vi "DriveExecute.vi"(8 "error in (no error)":errorcluster) -> (0 "error out":errorcluster)   [LabVIEW 2023]
doc: "Execute for Drie\n\nClosed control loop for drive\n\ninput: \n error in (cluster)\n\noutput:\n error out (cluster)"
uses:
  DriveGlobal.vi
  <vilib>/Rock Robotics/WPI/ThirdParty/JAS_Junk/TrajLib/Trajectory_Library.lvlib
  <vilib>/Rock Robotics/WPI/ThirdParty/JAS_Junk/TrajLib/LinearFilter_LP_BW1_Execute.vi
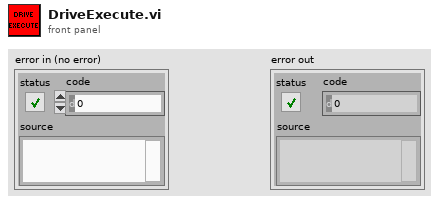
[diagram p1: front panel]
types:
  T1 = typedef "Trajectory_Library.lvlib/CHASSIS_SPEEDS.ctl" = cluster{"vX":dbl, "vY":dbl, "vOmega":dbl}
  T2 = typedef "ADIS16470 Device Reference.ctl" = cluster{"DevStatus":errorcluster, "Hardware Config":T3, "Calibration Complete":refnum<notifier>, "Status Reference":refnum<data-value>, "Data Reference":refnum<data-value>, "Sychronous Process VI":T7, "Cmd FIFO":refnum<k33>, "Source":T8, "Data FIFO":refnum<k33>, "Calibration Time (ms)":u32, "Data Reference":refnum<data-value>}
  T3 = typedef "ADIS16470 Hardware Configuration.ctl" = cluster{"SPI Clock Rate (Hz)":dbl, "IMU SPI Mode (3)":T4, "IMU Reset Pin":T5, "IMU SPI Bus":T6, "IMU Data Ready Pin":T5, "Stall Config":cluster{"Pow2BytesPerRead":u8, "StallTicks":u16, "CsToSclkTicks":u8}}
  T4 = typedef "WPI_SPIMode.ctl" = enum16{"Mode 0 (Clk Idle Low,Sample on Leading)", "Mode 1 (Clk Idle Low,Sample on Trailing)", "Mode 2 (Clk Idle High,Sample on Leading)", "Mode 3 (Clk Idle High,Sample on Trailing)"}
  T5 = typedef "FPGA_DIOChannel.ctl" = enum8{"DIO 0", "DIO 1", "DIO 2", "DIO 3", "DIO 4", "DIO 5", "DIO 6", "DIO 7", "DIO 8", "DIO 9", "DIO MXP 0", "DIO MXP 1", "DIO MXP 2", "DIO MXP 3", "DIO MXP 4", "DIO MXP 5", "DIO MXP 6", "DIO MXP 7", "DIO MXP 8", "DIO MXP 9", "DIO MXP 10", "DIO MXP 11", "DIO MXP 12", "DIO MXP 13", "DIO MXP 14", "DIO MXP 15", "SPI Port CS1", "SPI Port CS2", "SPI Port CS3", "SPI Port MISO", "SPI Port MOSI", "Invalid"}
  T6 = typedef "spi_bus.ctl" = enum16{"SPI On-Board, CS0", "SPI On-Board, CS1", "SPI On-Board, CS2", "SPI On-Board, CS3", "SPI MXP", "Invalid"}
  T7 = typedef "ADIS16470 Process.ctl" = refnum<vi>
  T8 = typedef "FPGA_CounterEncoderSourceConvertionLVSourceType.ctl" = cluster{"DevStatus":errorcluster, "AnalogTriggerMode?":bool, "DigitalMode":cluster{"DIO Channel":T9}, "AnalogTriggerMode":cluster{"AnalogTriggerIndex":T10, "OutputType":T11}}
  T9 = typedef "FPGA_DIODigitalSourceChannel.ctl" = enum8{"DIO 0", "DIO 1", "DIO 2", "DIO 3", "DIO 4", "DIO 5", "DIO 6", "DIO 7", "DIO 8", "DIO 9", "DIO MXP 0", "DIO MXP 1", "DIO MXP 2", "DIO MXP 3", "DIO MXP 4", "DIO MXP 5", "DIO MXP 6", "DIO MXP 7", "DIO MXP 8", "DIO MXP 9", "DIO MXP 10", "DIO MXP 11", "DIO MXP 12", "DIO MXP 13", "DIO MXP 14", "DIO MXP 15", "SPI Port CS1", "SPI Port CS2", "SPI Port CS3", "SPI Port MISO", "SPI Port MOSI", "Disabled"}
  T10 = typedef "FPGA_AnalogTriggerIndex.ctl" = enum8{"Trig 0", "Trig 1", "Trig 2", "Trig 3", "Trig 4", "Trig 5", "Trig 6", "Trig 7", "Invalid"}
  T11 = typedef "FPGA_AnalogTriggerOutType.ctl" = enum16{"InWindow", "TriggerState", "Rising", "Falling"}
  T12 = typedef "Trajectory_Library.lvlib/SWERVE_DRIVE_KINEMATICS.ctl" = cluster{"NumModules":i32, "InverseKinematics":T13, "ForwardKinematics":T13, "Modules":T14[], "PrevCoR":T14, "SavedModuleStates":T15[]}
  T13 = typedef "NI_Matrix.lvlib/RealMatrix.ctl" = dbl[][]
  T14 = typedef "Trajectory_Library.lvlib/TRANSLATION2D.ctl" = cluster{"X":dbl, "Y":dbl}
  T15 = typedef "Trajectory_Library.lvlib/SWERVE_DRIVE_MODULE_STATE.ctl" = cluster{"Speed":dbl, "Angle":T16}
  T16 = typedef "Trajectory_Library.lvlib/ROTATION2D.ctl" = cluster{"VALUE":dbl, "COS":dbl, "SIN":dbl}
  T17 = typedef "Trajectory_Library.lvlib/SWERVE_DRIVE_MODULE_POSITION.ctl" = cluster{"Distance":dbl, "Angle":T16, "P":bool}
  T18 = typedef "ADIS16470 Data.ctl" = cluster{"XAngle":dbl, "YAngle":dbl, "ZAngle":dbl}
  T19 = typedef "ADIS16470 Status.ctl" = cluster{"Calibrated?":bool, "IMU Detected?":bool}
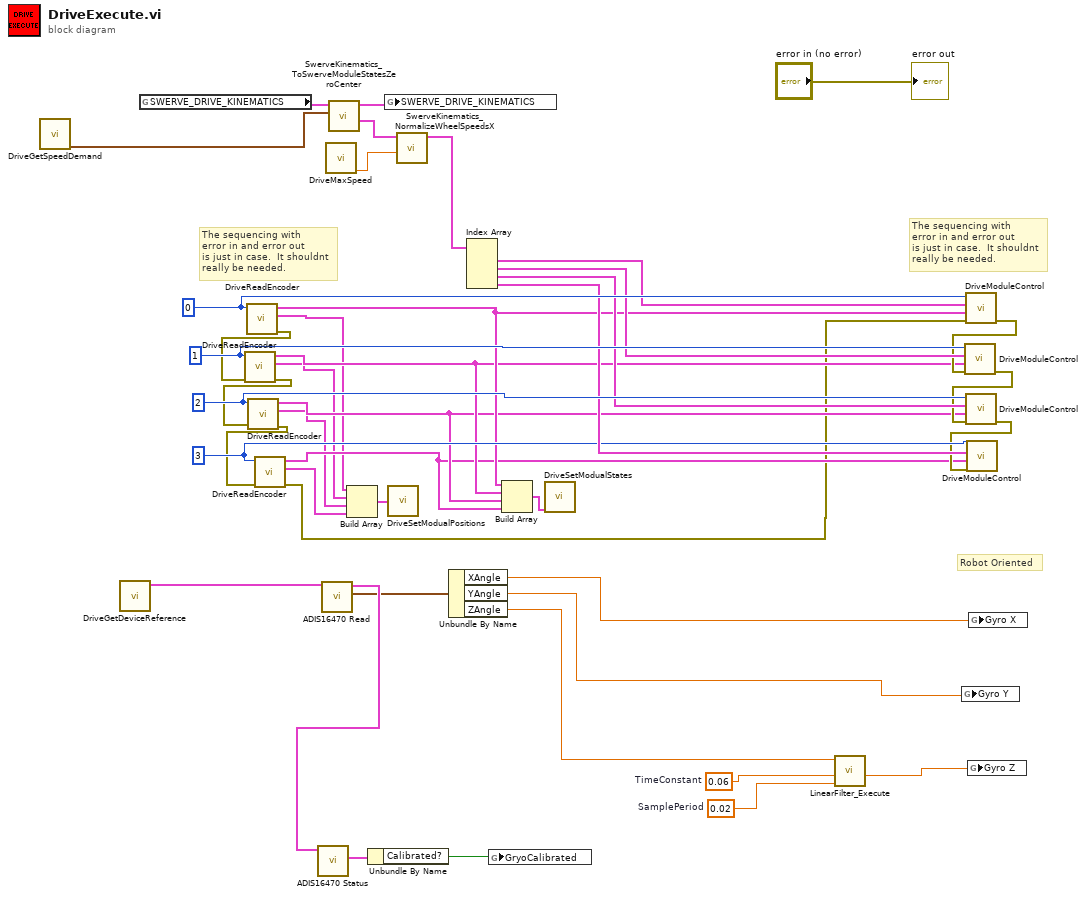
[diagram p0: block diagram]
diagram:
  w15 = 0.02  # SamplePeriod
  w1 = 0.06  # TimeConstant
  w39 = 0 ("ModualNamePrefix")
  w38 = 1 ("ModualNamePrefix")
  w37 = 2 ("ModualNamePrefix")
  w32 = 3 ("ModualNamePrefix")
  # "Robot Oriented"
  # "The sequencing with\nerror in and error out\nis just in case.  It shouldnt\nreally be needed."
  # "The sequencing with\nerror in and error out\nis just in case.  It shouldnt\nreally be needed."
  n1 = call "DriveGetSpeedDemand.vi"() -> ("ChassisSpeedDemand"=w41:T1)  [unwired: 8 in, 3 out]
  n2 = call "DriveGetDeviceReference.vi"() -> ("ADIS16470DevRef out"=w14:T2)  [unwired: 11 in]
  n3 = global read "DriveGlobal.vi" "SWERVE_DRIVE_KINEMATICS"() -> (w42:T12)
  n4 = call "DriveReadEncoder.vi"("ModualNamePrefix"=w39) -> ("error out"=w18:errorcluster, "SWERVE_DRIVE_MODULE_POSITION"=w24:T17, "SWERVE_DRIVE_MODULE_STATE"=w28:T15)  [unwired: 8 in]
  n5 = call "DriveReadEncoder.vi"("error in"=w18, "ModualNamePrefix"=w38) -> ("error out"=w17:errorcluster, "SWERVE_DRIVE_MODULE_POSITION"=w23:T17, "SWERVE_DRIVE_MODULE_STATE"=w27:T15)  [unwired: 7 in]
  n6 = call "DriveReadEncoder.vi"("error in"=w17, "ModualNamePrefix"=w37) -> ("error out"=w16:errorcluster, "SWERVE_DRIVE_MODULE_POSITION"=w22:T17, "SWERVE_DRIVE_MODULE_STATE"=w26:T15)  [unwired: 7 in]
  n7 = call "DriveReadEncoder.vi"("error in"=w16, "ModualNamePrefix"=w32) -> ("error out"=w5:errorcluster, "SWERVE_DRIVE_MODULE_POSITION"=w21:T17, "SWERVE_DRIVE_MODULE_STATE"=w25:T15)  [unwired: 7 in]
  n8 = call <vilib>:"ADIS16470 Read.vi"("ADIS16470DevRef"=w14) -> ("ADIS16470 Value"=w10:T18, "ADIS16470DevRef"=w11:T2)  [unwired: 7 in, 2 out]
  n9 = call <vilib>:"ADIS16470 Status.vi"("ADIS16470DevRef"=w11) -> ("ADIS16470 Status"=w13:T19)  [unwired: 8 in, 2 out]
  n10 = call "DriveMaxSpeed.vi"() -> ("Max Speed (m/sec)"=w3:dbl)  [unwired: 10 in, 1 out]
  n11 = call <vilib>:"SwerveKinematics_ToSwerveModuleStatesZeroCenter.vi"("ChassisSpeeds"=w41, "in SWERVE_DRIVE_KINEMATICS"=w42) -> ("ModuleStates"=w4:T15[], "out SWERVE_DRIVE_KINEMATICS"=w40:T12)  [unwired: 8 in]
  n12 = Build Array(w24, w23, w22, w21) -> (w19:T17[])
  n13 = Unbundle By Name(w13) -> ("Calibrated?"=w12:bool)
  n14 = global write "DriveGlobal.vi" "SWERVE_DRIVE_KINEMATICS"(w40) -> ()
  n15 = call "DriveSetModualPositions.vi"("Swerve_Drive_Modual_Position"=w19) -> ()  [unwired: 11 in]
  n16 = call <vilib>:"SwerveKinematics_NormalizeWheelSpeedsX.vi"("AttainableMaxSpeed"=w3, "in WheelStates"=w4) -> ("out WheelStates"=w2:T15[])  [unwired: 9 in]
  n17 = Unbundle By Name(w10) -> ("XAngle"=w8:dbl, "YAngle"=w7:dbl, "ZAngle"=w9:dbl)
  n18 = Index Array(array=w2) -> (element #1=w33:T15, element #2=w36:T15, element #3=w35:T15, element #4=w34:T15)  [unwired: 4 in]
  n19 = global write "DriveGlobal.vi" "GryoCalibrated"(w12) -> ()
  n20 = Build Array(w28, w27, w26, w25) -> (w20:T15[])
  n21 = call "DriveSetModualStates.vi"("Swerve__Drive_Modual_States"=w20) -> ()  [unwired: 11 in]
  n22 = call-poly <vilib>:"LinearFilter_Execute.vi"("SamplePeriod"=w15, "TimeConstant"=w1, "Input"=w9) -> ("Output"=w6:dbl)  [unwired: 8 in]
  n23 = global write "DriveGlobal.vi" "Gyro Y"(w7) -> ()
  n24 = call "DriveModuleControl.vi"("error in"=w5, "Actual State"=w28, "Desired State"=w33, "ModualNamePrefix"=w39) -> ("error out"=w31:errorcluster)  [unwired: 7 in]
  n25 = call "DriveModuleControl.vi"("error in"=w31, "Actual State"=w27, "Desired State"=w36, "ModualNamePrefix"=w38) -> ("error out"=w30:errorcluster)  [unwired: 7 in]
  n26 = call "DriveModuleControl.vi"("error in"=w30, "Actual State"=w26, "Desired State"=w35, "ModualNamePrefix"=w37) -> ("error out"=w29:errorcluster)  [unwired: 7 in]
  n27 = call "DriveModuleControl.vi"("error in"=w29, "Actual State"=w25, "Desired State"=w34, "ModualNamePrefix"=w32) -> ()  [unwired: 7 in, 1 out]
  n28 = global write "DriveGlobal.vi" "Gyro Z"(w6) -> ()
  n29 = global write "DriveGlobal.vi" "Gyro X"(w8) -> ()
  "error out" <- "error in (no error)"
